vi "bats.parser.test.vi"() -> ()   [LabVIEW 2020]
uses:
  <vilib>/Platform/TimedLoop/XDataNode/timing_clust.ctl
  <vilib>/Platform/TimedLoop/XDataNode/nitl_modes.ctl
  <vilib>/Platform/TimedLoop/XDataNode/wakeup.ctl
  Test/test.data.in.ctl
  <vilib>/rvi/DataTransferAndStorage/Container/Common/niFpgaContainerGetUniqueNameForEmu.vi
  <vilib>/rvi/DataTransferAndStorage/Container/Common/niFpgaContainerSetEmuInfo.vi
  <vilib>/rvi/eio/common/nirviEmuReportErrorAndStop.vi
  <vilib>/rvi/Emulation/niFpgaSctlEmulationGetInTimedLoop.vi
  <vilib>/rvi/Emulation/niFpgaEmulationReportErrorSimple.vi
  <vilib>/rvi/Emulation/niFpgaGetClockAttributes.vi
  <vilib>/rvi/Emulation/niFpgaCriticalErrorInLSC.vi
  <vilib>/rvi/interface/RandomDataEmulation/niFpgaRandomDataHandleErrors.vi
  <vilib>/rvi/DataTransferAndStorage/Container/Common/niFpgaContainerExecOnDevCompGetState.vi
  <vilib>/rvi/Emulation/niFpgaEmulationIsFPGAContextNoSignature.vi
  <vilib>/rvi/errors/niFpgaSetErrorForExecOnDevCompSimple.vi
  <vilib>/rvi/FIFO/Fifo_Resource/nirvififoEmulationSetSize.vi
  <vilib>/rvi/FIFO/Fifo_Resource/nirviFifoEmulationQueueMgr.vi
  <instcachedir>/0/nirviFifoEmulationQueueMgr_E5CAEC123FF24DC58D834DCA3CDAA9B5.lvgen/nirviFifoEmulationQueueMgr_E5CAEC123FF24DC58D834DCA3CDAA9B5_003.vi
  <vilib>/rvi/FIFO/Fifo_Resource/nirvififoEmulationDetermineInputValidOut.vi
  <vilib>/rvi/FIFO/Fifo_Resource/nirvififoEmulationCreateLock.vi
  <vilib>/rvi/Emulation/niFpgaProcessEmulError.vi
  <vilib>/rvi/FIFO/Fifo_Resource/nirvififoEmulationObtainLock.vi
  <vilib>/rvi/FIFO/Fifo_Resource/nirvififoEmulationReleaseLock.vi
  <vilib>/rvi/occurrence/nirviWaitOnOccurrenceBase.vi
  <vilib>/rvi/errors/nirviReportUnexpectedCaseInternalError.vi
  <vilib>/rvi/errors/nirviReportUnexpectedCaseInternalError (U32).vi
  <vilib>/Utility/error.llb/Clear Errors.vi
  <instcachedir>/0/nirviFifoEmulationQueueMgr_E5CAEC123FF24DC58D834DCA3CDAA9B5.lvgen/nirviFifoEmulationQueueMgr_E5CAEC123FF24DC58D834DCA3CDAA9B5_001.vi
  <vilib>/rvi/interface/RandomDataEmulation/nirviRandomDataMultiElementFPGAFIFO.vi
  <instcachedir>/0/nirviRandomDataMultiElementFPGAFIFO_3E9965BA1FAD4E7B8DABA31768A09B1F.lvgen/nirviRandomDataMultiElementFPGAFIFO_3E9965BA1FAD4E7B8DABA31768A09B1F_000.vi
  <vilib>/Platform/TimedLoop/XDataNode/XDataNode.xnode
  <vilib>/rvi/LocalResourceManager/LocalResourceManager.xnode
  <vilib>/rvi/DataTransferAndStorage/Container/XNode/niFpgaContainer.xnode
  <vilib>/rvi/interface/RandomDataEmulation/nirviRandomDataFpgaReadWriteTemplate.vi
  <vilib>/rvi/FIFO/Fifo_Resource/niFpgaFifoEmulationRefIn.vi
  <vilib>/rvi/FIFO/Fifo_Resource/nirvififoEmulationRead.vi
  <vilib>/rvi/interface/RandomDataEmulation/nirviRandomDataFpgaMultiElementTemplate.vi
  <vilib>/Platform/TimedLoop/XDataNode/XDNodeRunTimeDep.lvlib
panel:
  in  "reset":bool
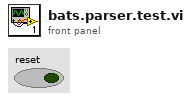
[diagram p1: front panel]
types:
  T1 = typedef "XDNodeRunTimeDep.lvlib/timing_clust.ctl" = cluster{"Expected End [f-1]":u64, "Actual End [f-1]":u64, "Finished Late? [f-1]":bool, "Expected End [i-1]":u64, "Actual End [i-1]":u64, "Finished Late? [i-1]":bool, "Expected Start [i]":u64, "Actual Start [i]":u64, "Expected Start [f]":u64, "Actual Start [f]":u64, "Source Name":string, "Structure Name":string, "Period":i64, "Deadline":i64, "Offset":i64, "Start":i64, "Priority":i32, "Timeout":i32, "Mode":T2, "Wakeup Reason":T3, "Error":errorcluster, "Source Type":string, "Secondary Source Type":string, "Global End Time":u64, "Global Start Time":u64, "Frame Duration":u64, "Iteration Duration":u64, "Assigned CPU":i32, "I/O Scan Engine Mode":u32}
  T2 = typedef "XDNodeRunTimeDep.lvlib/nitl_modes.ctl" = enum32{"No Change", "Process missed periods, maintain original phase", "Discard missed periods, maintain original phase", "Process missed periods, ignore original phase", "Discard missed periods, ignore original phase"}
  T3 = typedef "XDNodeRunTimeDep.lvlib/wakeup.ctl" = enum32{"Normal", "Aborted", "Asynchronous wakeup", "Timing source error", "Timed loop error", "Timeout"}
  T4 = cluster{"OrderBook Command.Type":enum16{"AddOrder", "OrderExecuted", "ReduceSize", "ModifyOrder", "DeleteOrder", "Get.All.Orders", "Get.Top"}, "Side (U8)":u8, "Order Id (U64)":u64, "Quantity (U32)":u32, "Symbol (U64)":u64, "Price (U64)":u64, "Executed Quantity (U32)":u32, "Cancelled Quantity (U32)":u32}
  T5 = enum16{"AddOrder", "OrderExecuted", "ReduceSize", "ModifyOrder", "DeleteOrder", "Get.All.Orders", "Get.Top"}
  T6 = typedef "test.data.in.ctl" = cluster{"data":u8, "end_of_frame":bool}
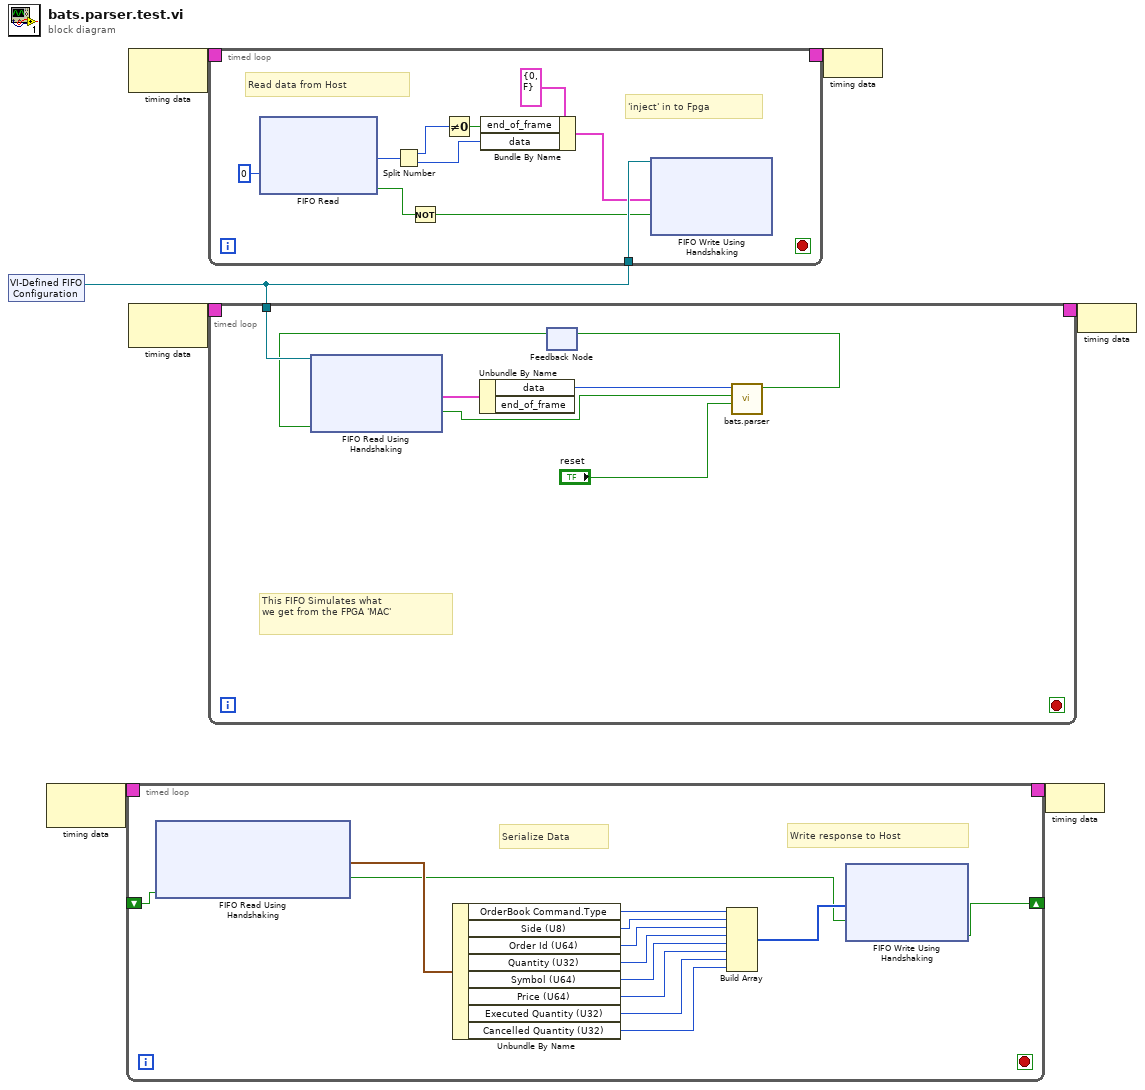
[diagram p0: block diagram]
diagram:
  n1 = xnode "VI-Defined FIFO Configuration"() -> ("FIFO Out"=w3:refnum<k21>)
  n2 = node-c288() -> (w2:T1)  [unwired: 1 in]
  n3 = timed-loop {
    timing: w2 -> [_]
    timing-out: [_] -> w1
    shift-right: [w20] -> _
    shift-left: _ -> [w10]
    stop <- _ stop-if-true
    # "Serialize Data"
    # "Write response to Host"
    n4 = xnode "FIFO Read Using Handshaking"("Ready for Output"=w10) -> ("Element"=w9:T4, "Output Valid"=w8:bool)  [unwired: 1 in, 1 out]
    n5 = Unbundle By Name(w9) -> ("OrderBook Command.Type"=w19:T5, "Side (U8)"=w18:u8, "Order Id (U64)"=w17:u64, "Quantity (U32)"=w16:u32, "Symbol (U64)"=w15:u64, "Price (U64)"=w14:u64, "Executed Quantity (U32)"=w13:u32, "Cancelled Quantity (U32)"=w12:u32)
    n6 = Build Array(w19, w18, w17, w16, w15, w14, w13, w12) -> (w11:u64[])
    n7 = xnode "FIFO Write Using Handshaking"("Element"=w11, "Input Valid"=w8) -> ("Ready for Input"=w20:bool)  [unwired: 1 in, 1 out]
  }
  n8 = node-c288() -> (w7:T1)  [unwired: 1 in]
  n9 = node-c288() -> (w5:T1)  [unwired: 1 in]
  n10 = timed-loop {
    timing: w7 -> [_]
    timing-out: [_] -> w6
    tunnel: w3 -> [w32]
    stop <- _ stop-if-true
    # "'inject' in to Fpga"
    # "Read data from Host"
    n11 = xnode "FIFO Read"("Timeout"=0) -> ("Element"=w28:u64, "Timed Out?"=w30:bool)  [unwired: 1 in, 1 out]
    n12 = Split Number(x=w28) -> (hi(x)=w24:u32, lo(x)=w26:u32)
    n13 = Not(x=w30) -> (.not. x?=w29:bool)
    n14 = Not Equal To 0?(x=w24) -> (x != 0?=w25:bool)
    n15 = Bundle By Name(cluster=T6 {"data"=0, "end_of_frame"=FALSE} ("Cluster"), "end_of_frame"=w25, "data"=w26) -> (w23:T6)
    n16 = xnode "FIFO Write Using Handshaking"("Element"=w23, "Input Valid"=w29, "FIFO In"=w32) -> ()  [unwired: 2 out]
  }
  n17 = timed-loop {
    timing: w5 -> [_]
    timing-out: [_] -> w4
    tunnel: w3 -> [w41]
    stop <- _ stop-if-true
    # "This FIFO Simulates what\nwe get from the FPGA 'MAC'"
    n18 = feedback #1() -> (w35:bool)  [unwired: 1 in]
    n19 = xnode "FIFO Read Using Handshaking"("Ready for Output"=w35, "FIFO In"=w41) -> ("Element"=w40:cluster{"data":u8, "end_of_frame":bool}, "Output Valid"=w37:bool)  [unwired: 1 out]
    n20 = Unbundle By Name(w40) -> ("data"=w39:u8)  [unwired: 1 out]
    n21 = call "bats.parser.vi"("reset"="reset", "data_valid"=w37, "data"=w39) -> ("Ready.for.Udp.Input"=w36:bool)  [unwired: 8 in]
    n22 = feedback-in #1(w36) -> ()
  }
  n23 = node-c288(w6) -> ()
  n24 = node-c288(w1) -> ()
  n25 = node-c288(w4) -> ()
